vi "Unit Test Mutation (Nested Typedefs).vi"() -> ()   [LabVIEW 2019, in "Sports Unit Tests.lvclass"]
uses:
  Sports Unit Tests.lvclass
  Classes/Kobe Bryant/Kobe Bryant.lvclass
  <vilib>/Utility/error.llb/Clear Errors.vi
  <vilib>/addons/_JKI Toolkits/Caraya/classes/Test/Define Test.vi
  <vilib>/addons/_JKI Toolkits/Caraya/classes/Assert/Assert Equal Value_Variant.vi
  <vilib>/addons/_JKI Toolkits/Caraya/classes/Assert/Assert Not Error.vi
  <vilib>/addons/_JKI Toolkits/Caraya/classes/Assert/Assert.lvclass
  Classes/Kobe Bryant/KobeData2.ctl
  Classes/Kobe Bryant/KobeEnum.ctl
  Classes/Kobe Bryant/KobeData1.ctl
  <userlib>/Blue Origin/BlueSerialization/BlueSerializer/BlueSerializer.lvclass
panel:
  out "Table":string[][](table)=[["{\r  \"Class\":[\"Kobe Bryant.lvclass\",\"Basketball Player.lvclass\",\"Sports Player.lvclass\",\"Human.lvclass\",\"BlueSerialization.lvlib:BlueSerializable.lvclass\"],\r  \"Version\":[\"2.0.0.3\",\"2.0.0.3\",\"2.0.0.3\",\"2.0.0.3\",\"2.0.0.0\"],\r  \"BlueSerialization.lvlib:BlueSerializable.lvclass\":{\"LibVersion\":1},\r  \"Human.lvclass\":{\r    \"alive?\":false,\r    \"Age (years)\":40,\r    \"Name\":\"KobeBryant\",\r    \"Height (ft)\":6\r  },\r  \"Sports Player.lvclass\":{\r    \"Professional?\":true,\r    \"Earnings (dollars)\":1000000,\r    \"Sponsor\":\"Additas\"\r  },\r  \"Basketball Player.lvclass\":{\r    \"Sports team\":\"Lakers\",\r    \"Free-throw percentage\":70\r  },\r  \"Kobe Bryant.lvclass\":{\r    \"Typedefs\":{\r      \"Kobenumber\":123,\r      \"KobeBool\":true,\r      \"KobeSubTpyedef\":{\"KobeString\":\"hello\",\"KobeNumber\":3.14},\r      \"KobeEnum\":\"a\"\r    },\r    \"Numeric\":0\r  }\r}", "{\r  \"Class\":[\"Kobe Bryant.lvclass\",\"Basketball Player.lvclass\",\"Sports Player.lvclass\",\"Human.lvclass\",\"BlueSerialization.lvlib:BlueSerializable.lvclass\"],\r  \"Version\":[\"2.0.0.3\",\"2.0.0.3\",\"2.0.0.3\",\"2.0.0.3\",\"2.0.0.0\"],\r  \"BlueSerialization.lvlib:BlueSerializable.lvclass\":{\"LibVersion\":1},\r  \"Human.lvclass\":{\r    \"alive?\":false,\r    \"Age (years)\":40,\r    \"Name\":\"KobeBryant\",\r    \"Height (ft)\":6\r  },\r  \"Sports Player.lvclass\":{\r    \"Professional?\":true,\r    \"Earnings (dollars)\":1000000,\r    \"Sponsor\":\"Additas\"\r  },\r  \"Basketball Player.lvclass\":{\r    \"Sports team\":\"Lakers\",\r    \"Free-throw percentage\":70\r  },\r  \"Kobe Bryant.lvclass\":{\r    \"Typedefs\":{\r      \"Kobenumber\":123,\r      \"KobeBool\":true,\r      \"KobeSubTpyedef\":{\"KobeString\":\"hello\",\"KobeNumber\":3.14},\r      \"KobeEnum\":\"a\"\r    },\r    \"Numeric\":0\r  }\r}", "Status: FALSE\ncode: 0\n", "BlueJSONTextSerializer.lvlib:BlueJSONTextSerializer.lvclass"], ["Class = [\"Kobe Bryant.lvclass\", \"Basketball Player.lvclass\", \"Sports Player.lvclass\", \"Human.lvclass\", \"BlueSerialization.lvlib:BlueSerializable.lvclass\"]\r\nVersion = [\"2.0.0.3\", \"2.0.0.3\", \"2.0.0.3\", \"2.0.0.3\", \"2.0.0.0\"]\r\n\n[\"BlueSerialization.lvlib:BlueSerializable.lvclass\"]\nLibVersion = 1\r\n\n[\"Human.lvclass\"]\n\"alive?\" = false\r\n\"Age (years)\" = 40\r\nName = \"KobeBryant\"\r\n\"Height (ft)\" = 6.0\r\n\n[\"Sports Player.lvclass\"]\n\"Professional?\" = true\r\n\"Earnings (dollars)\" = 1000000.0\r\nSponsor = \"Additas\"\r\n\n[\"Basketball Player.lvclass\"]\n\"Sports team\" = \"Lakers\"\r\n\"Free-throw percentage\" = 70.0\r\n\n[\"Kobe Bryant.lvclass\"]\nNumeric = 0.0\r\n\n[\"Kobe Bryant.lvclass\".Typedefs]\nKobenumber = 123.0\r\nKobeBool = true\r\nKobeEnum = \"a\"\r\n\n[\"Kobe Bryant.lvclass\".Typedefs.KobeSubTpyedef]\nKobeString = \"hello\"\r\nKobeNumber = 3.14\r\n", "Class = [\"Kobe Bryant.lvclass\", \"Basketball Player.lvclass\", \"Sports Player.lvclass\", \"Human.lvclass\", \"BlueSerialization.lvlib:BlueSerializable.lvclass\"]\r\nVersion = [\"2.0.0.3\", \"2.0.0.3\", \"2.0.0.3\", \"2.0.0.3\", \"2.0.0.0\"]\r\n\n[\"BlueSerialization.lvlib:BlueSerializable.lvclass\"]\nLibVersion = 1\r\n\n[\"Human.lvclass\"]\n\"alive?\" = false\r\n\"Age (years)\" = 40\r\nName = \"KobeBryant\"\r\n\"Height (ft)\" = 6.0\r\n\n[\"Sports Player.lvclass\"]\n\"Professional?\" = true\r\n\"Earnings (dollars)\" = 1000000.0\r\nSponsor = \"Additas\"\r\n\n[\"Basketball Player.lvclass\"]\n\"Sports team\" = \"Lakers\"\r\n\"Free-throw percentage\" = 70.0\r\n\n[\"Kobe Bryant.lvclass\"]\nNumeric = 0.0\r\n\n[\"Kobe Bryant.lvclass\".Typedefs]\nKobenumber = 123.0\r\nKobeBool = true\r\nKobeEnum = \"a\"\r\n\n[\"Kobe Bryant.lvclass\".Typedefs.KobeSubTpyedef]\nKobeString = \"hello\"\r\nKobeNumber = 3.14\r\n", "Status: FALSE\ncode: 0\n", "BlueTOMLSerializer.lvlib:BlueTOMLSerializer.lvclass"]]
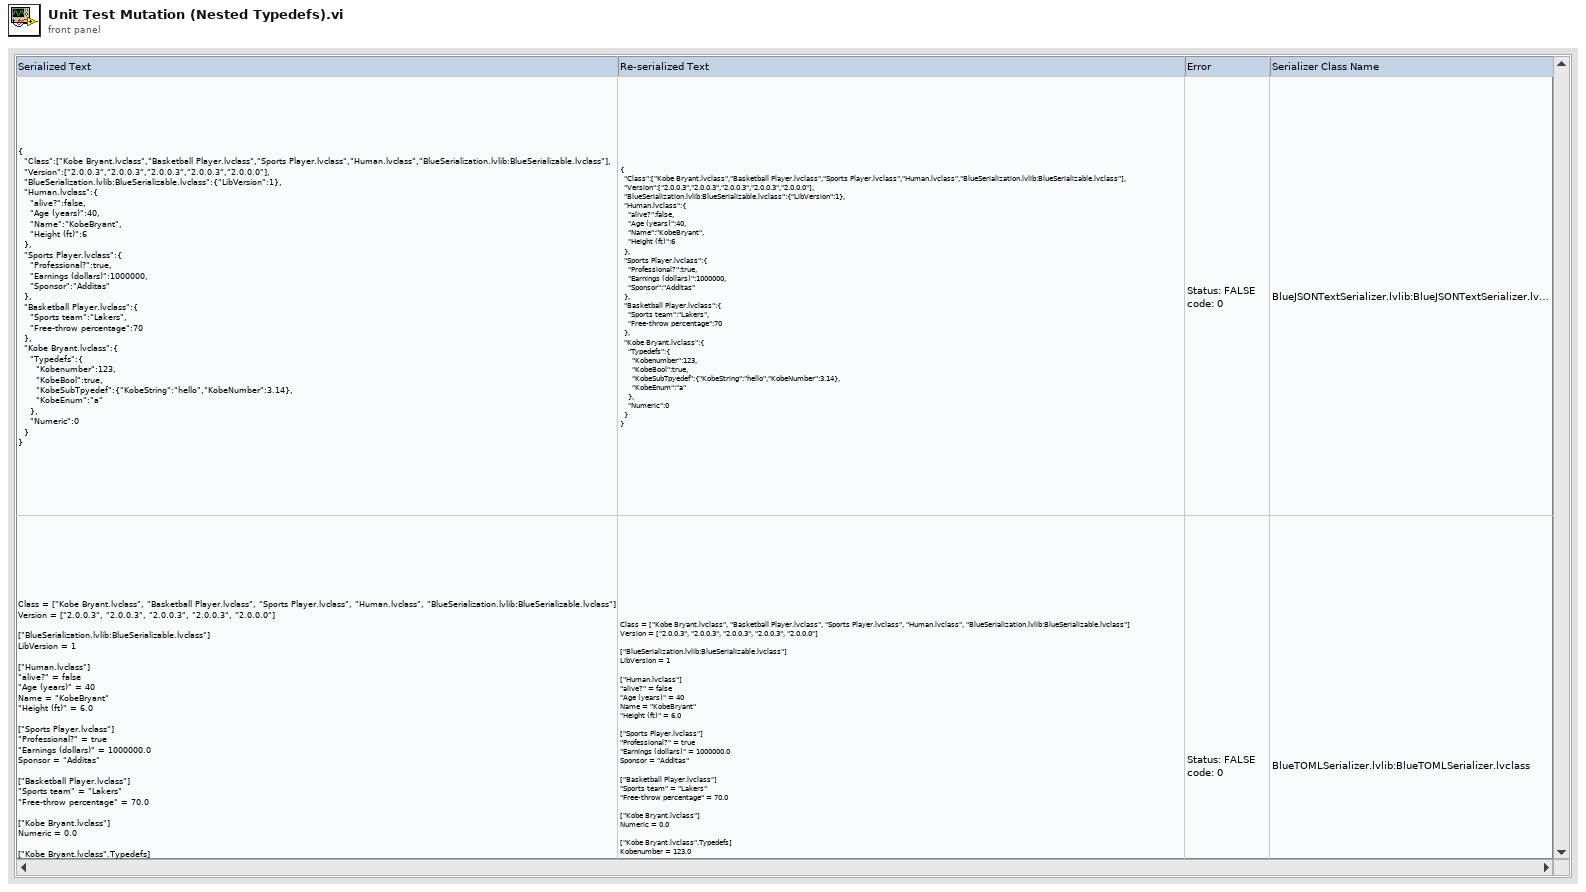
[diagram p1: front panel]
types:
  T1 = typedef "Kobe Bryant.lvclass/KobeData1.ctl" = cluster{"Kobenumber":dbl, "KobeBool":bool, "KobeSubTpyedef":T2, "KobeEnum":T3}
  T2 = typedef "Kobe Bryant.lvclass/KobeData2.ctl" = cluster{"KobeString":string, "KobeNumber":dbl}
  T3 = typedef "Kobe Bryant.lvclass/KobeEnum.ctl" = enum16{"1", "2", "3", "4", "5"}
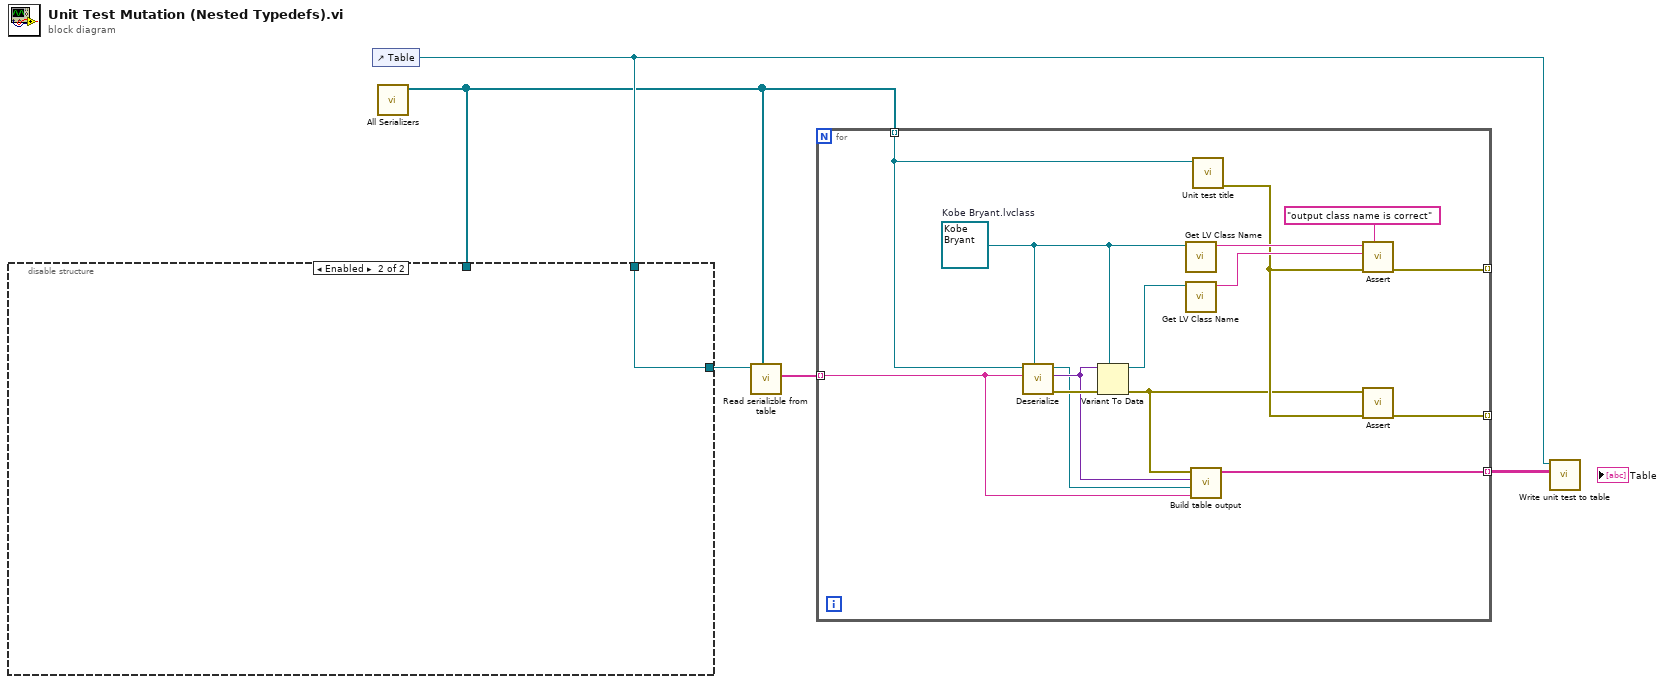
[diagram p0: block diagram]
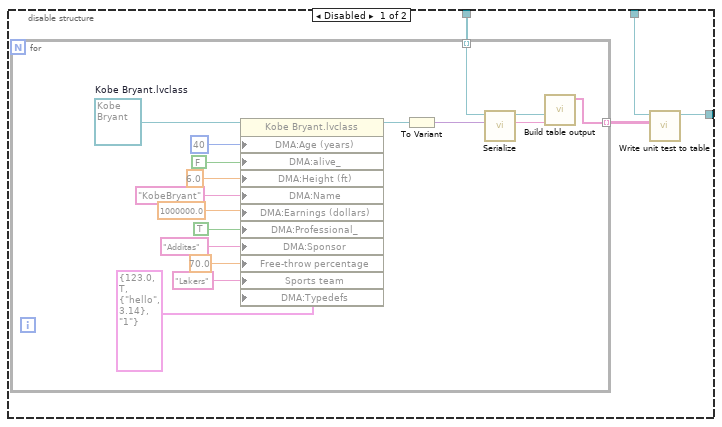
[diagram p2: hidden frame]
diagram:
  n1 = control-ref of="Table"() -> (w5:refnum<vi>)
  n2 = call "All Serializers.vi"() -> ("All serializers"=w2:refnum<class "BlueSerializer.lvclass">[])  [unwired: 11 in]
  n3 = disable-structure shown="Enabled" {
    disable-tunnel: w5 -> [w8 w27]
    disable-tunnel: [w7 w27] -> w4
    disable-tunnel: w2 -> [w6 _]
    frame Disabled {
      n4 = for {
        tunnel: w6 -> [w17] mode=indexing
        tunnel: [w14] -> w9 mode=indexing
        w13 = refnum<class "Kobe Bryant.lvclass"> refnum  # Kobe Bryant.lvclass
        n5 = property on="Property Node" class="Kobe Bryant.lvclass"(reference=w13, "DMA:Age (years)"=u16 40 ("Age (years)"), "DMA:alive_"=FALSE ("alive_"), "DMA:Height (ft)"=6.0 ("Height (ft)"), "DMA:Name"="KobeBryant" ("Name"), "DMA:Earnings (dollars)"=1000000.0 ("Earnings (dollars)"), "DMA:Professional_"=TRUE ("Professional_"), "DMA:Sponsor"="Additas" ("Sponsor"), "Free-throw percentage"=70.0, "Sports team"="Lakers", "DMA:Typedefs"=T1 {"Kobenumber"=123.0, "KobeBool"=TRUE, "KobeSubTpyedef"={"KobeString"="hello", "KobeNumber"=3.14}, "KobeEnum"=enum."1"} ("Typedefs")) -> (reference out=w26:refnum<class "Kobe Bryant.lvclass">)  [unwired: 1 in, 1 out]
        n6 = To Variant(anything=w26) -> (Variant=w18:variant)
        n7 = call <userlib>:"Serialize.vi"("Anything"=w18, "BlueSerializer in"=w17) -> ("Serialized Text"=w16:string, "BlueSerializer out"=w15:refnum<class "BlueSerializer.lvclass">)  [unwired: 7 in, 1 out]
        n8 = call "Build table output.vi"("serialized text"=w16, "BlueSerializer in"=w15) -> ("table output"=w14:string[])  [unwired: 9 in]
      }
      n9 = call "Write unit test to table.vi"("Table"=w9, "Table ref in"=w8) -> ("Table ref out"=w7:refnum<vi>)  [unwired: 9 in]
    }
    frame Enabled {
    }
  }
  n10 = call "Read serializble from table.vi"("serializers"=w2, "Table ref in"=w4) -> ("serializable texts"=w3:string[])  [unwired: 7 in, 2 out]
  n11 = for {
    tunnel: w2 -> [w29] mode=indexing
    tunnel: [w37] -> _ mode=indexing
    tunnel: [w36] -> _ mode=indexing
    tunnel: w3 -> [w31] mode=indexing
    tunnel: [w30] -> w1 mode=indexing
    w28 = refnum<class "Kobe Bryant.lvclass"> refnum  # Kobe Bryant.lvclass
    n12 = call <userlib>:"Deserialize.vi"("Anything"=w28, "Serialized Text"=w31, "BlueSerializer in"=w29) -> ("error out"=w42:errorcluster, "Variant"=w33:variant, "BlueSerializer out"=w32:refnum<class "BlueSerializer.lvclass">)  [unwired: 6 in]
    n13 = Variant To Data(error in=w42, type=w28, Variant=w33) -> (data=w41:refnum<class "Kobe Bryant.lvclass">, error out=w34:errorcluster)
    n14 = call <vilib>:"Get LV Class Name.vi"("object"=w28) -> ("class name"=w40:string)  [unwired: 9 in, 1 out]
    n15 = call <vilib>:"Get LV Class Name.vi"("object"=w41) -> ("class name"=w39:string)  [unwired: 9 in, 1 out]
    n16 = call "Build table output.vi"("serialized text"=w31, "BlueSerializer in"=w32, "deserialized variant"=w33, "variant to data error"=w34) -> ("table output"=w30:string[])  [unwired: 7 in]
    n17 = call "Unit test title.vi"("serializer"=w29) -> ("error out"=w35:errorcluster)  [unwired: 9 in, 1 out]
    n18 = call-poly <vilib>:"Assert.vi"("Label"="output class name is correct", "error in (no error)"=w35, "Y"=w39, "X"=w40) -> ("error out"=w36:errorcluster)  [unwired: 7 in]
    n19 = call-poly <vilib>:"Assert.vi"("error in (no error)"=w35, "Not Error?"=w34) -> ("error out"=w37:errorcluster)  [unwired: 9 in]
  }
  n20 = call "Write unit test to table.vi"("Table"=w1, "Table ref in"=w5) -> ()  [unwired: 9 in, 1 out]
